vi "construct lorentzian.vi"(10 "omega  in":dbl[](array[numeric]), 11 "lorentzian":T1={"Amplitude"=-1.0311345636926572, "omega(0)"=-1.0311345636926572, "Gamma"=-1.0311345636926572, "phase"=-1.0311345636926572, "Q"=-1.0311345636926572, "Norm  Ampl"=-1.0311345636926572, "z (inf)"=-1.0311345636926572+0.0i, "4corners"={"z (-pi/2)"=-1.0311345636926572+0.5736824521422934i, "z(inf)"=-0.5200164984937075+1.0975277942502903i, "z (pi/2)"=-1.0311345636926572+0.5736824521422934i, "z center"=-0.5136528600391839+0.580046090596817i, "z(0)"=-0.5200164984937075+1.0975277942502903i, "radius"=-1.0311345636926572}} {"z (inf)" format="%#9_9f"; "Q" format="%#9_9f"; "phase" format="%#9_9f"; "Gamma" format="%#9_9f"; "omega(0)" format="%#9_9f"}) -> (2 "omega  out":dbl[](array[numeric]), 3 "z out":cdb[](array[numeric]))   [LabVIEW 2015]
uses:
  lorentzian.ctl
  circle corners.ctl
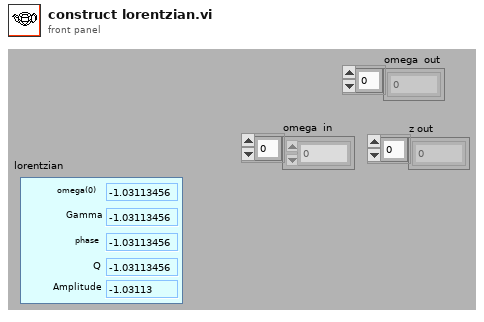
[diagram p1: front panel]
types:
  T1 = typedef "lorentzian.ctl" = cluster{"Amplitude":dbl, "omega(0)":dbl, "Gamma":dbl, "phase":dbl, "Q":dbl, "Norm  Ampl":dbl, "z (inf)":cdb, "4corners":T2}
  T2 = typedef "circle corners.ctl" = cluster{"z (-pi/2)":cdb, "z(inf)":cdb, "z (pi/2)":cdb, "z center":cdb, "z(0)":cdb, "radius":dbl}
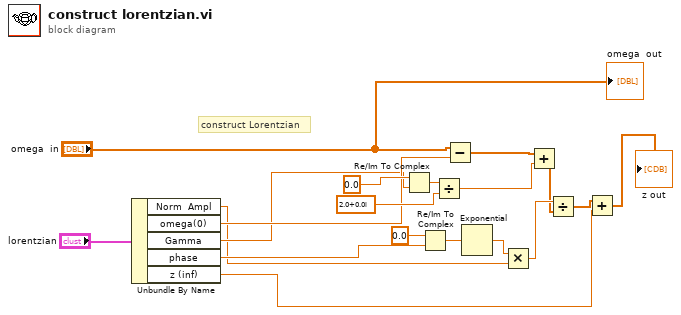
[diagram p0: block diagram]
diagram:
  # "construct Lorentzian"
  n1 = Unbundle By Name("lorentzian") -> ("Norm  Ampl"=w5:dbl, "omega(0)"=w8:dbl, "Gamma"=w7:dbl, "phase"=w6:dbl, "z (inf)"=w1:cdb)
  n2 = Re/Im To Complex(1:w7, 2:0.0 ("x")) -> (0:w13:cdb)
  n3 = Re/Im To Complex(1:w6, 2:0.0 ("x")) -> (0:w18:cdb)
  n4 = Divide(x=w13, y=cdb 2.0+0.0i) -> (x/y=w11:cdb)
  n5 = Subtract(x="omega  in", y=w8) -> (x-y=w15:dbl[])
  n6 = Exponential(1:w18) -> (0:w17:cdb)
  n7 = Multiply(x=w17, y=w5) -> (x*y=w16:cdb)
  n8 = Add(x=w15, y=w11) -> (x+y=w10:cdb[])
  n9 = Divide(x=w16, y=w10) -> (x/y=w9:cdb[])
  n10 = Add(x=w9, y=w1) -> (x+y=→"z out":cdb[])
  "omega  out" <- "omega  in"
